vi "concatenate.vi"(7 "images are appended as...":T1=enum."copy", 8 "error in (no error)":errorcluster, 10 "collection to append":refnum<class "ImageCollection.lvclass">, 11 "ImageCollection in":refnum<class "ImageCollection.lvclass">) -> (0 "error out":errorcluster, 3 "ImageCollection out":refnum<class "ImageCollection.lvclass">)   [LabVIEW 2010, in "ImageCollection.lvclass"]
uses:
  ImageCollection.lvclass
  add_mode_enum.ctl
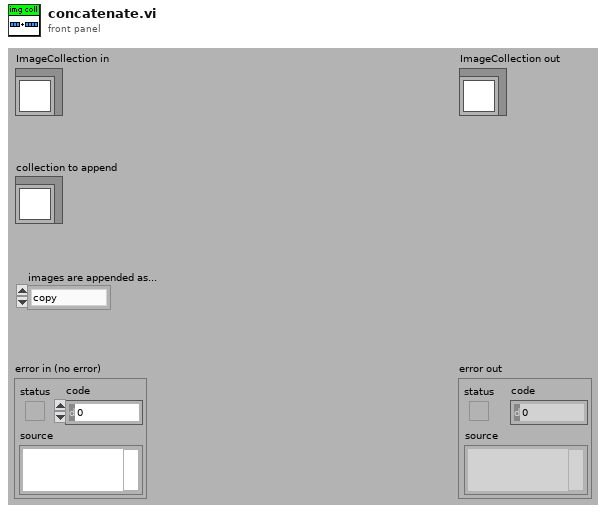
[diagram p1: front panel]
types:
  T1 = typedef "ImageCollection.lvclass/add_mode_enum.ctl" = enum16{"instance", "copy"}
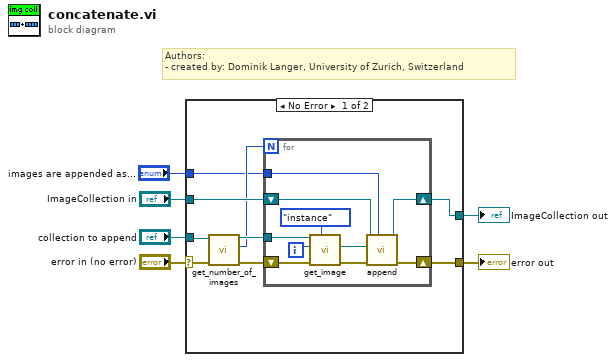
[diagram p0: block diagram]
diagram:
  # "Authors: \n- created by: Dominik Langer, University of Zurich, Switzerland"
  n1 = case shown="No Error" "error in (no error)" {
    selector: "error in (no error)" -> [w8 w27]
    tunnel: [w13 w27] -> w5
    tunnel: [w14 w26] -> w3
    tunnel: "ImageCollection in" -> [w15 w26]
    tunnel: "collection to append" -> [w7 _]
    tunnel: "images are appended as..." -> [w9 _]
    frame No Error {
      n2 = call-dynamic "get_number_of_images.vi"("error in (no error)"=w8, "ImageCollection in"=w7) -> ("error out"=w12:errorcluster, "size"=w10:i32, "ImageCollection out"=w11:refnum<class "ImageCollection.lvclass">)  [unwired: 7 out]
      n3 = for {
        N: w10 -> [_]
        tunnel: w11 -> [w23]
        shift-right: [w21] -> w13
        shift-left: w12 -> [w25]
        tunnel: w9 -> [w19]
        shift-right: [w17] -> w14
        shift-left: w15 -> [w22]
        i -> [w18]
        n4 = call-dynamic "get_image.vi"("get image as..."=add_mode_enum."instance", "error in (no error)"=w25, "index"=w18, "ImageCollection in"=w23) -> ("error out"=w24:errorcluster, "Image.lvclass"=w16:refnum<class "Image.lvclass">)  [unwired: 6 out]
        n5 = call-dynamic "append.vi"("add mode"=w19, "error in (no error)"=w24, "Image.lvclass"=w16, "ImageCollection in"=w22) -> ("error out"=w21:errorcluster, "ImageCollection out"=w17:refnum<class "ImageCollection.lvclass">)  [unwired: 6 out]
      }
    }
    frame Error {
    }
  }
  "error out" <- w5
  "ImageCollection out" <- w3
